vi "DSF.Execution.Runtime.Plugin Manager.Find Plugin Classes.Configuration.vi"(8 "error in (no error)":errorcluster, 10 "Plugin objects":refnum<class>[](array[class]), 11 "Plugin Manager in":refnum<class "DSF.Engine.Runtime.Plugin Manager.lvclass">) -> (0 "error out":errorcluster, 2 "Plugin Configuration Classes":T1, 3 "Plugin Manager out":refnum<class "DSF.Engine.Runtime.Plugin Manager.lvclass">)   [LabVIEW 2016, in "DSF.Engine.lvlib" / "DSF.Engine.Runtime.Plugin Manager.lvclass"]
uses:
  DSF.Engine.Runtime.Plugin Manager.lvclass
  Shared/Typedefs/DSF.Shared.Typedefs.Plugin Classes.Configuration.ctl
  Shared/Classes/Plugin/DSF.Shared.Configuration.Plugin.lvclass
  Shared/Classes/Transfer Group/DSF.Shared.Configuration.Transfer Group.lvclass
  Shared/Classes/Transfer/DSF.Shared.Configuration.Transfer.lvclass
  DSF.Shared.lvlib
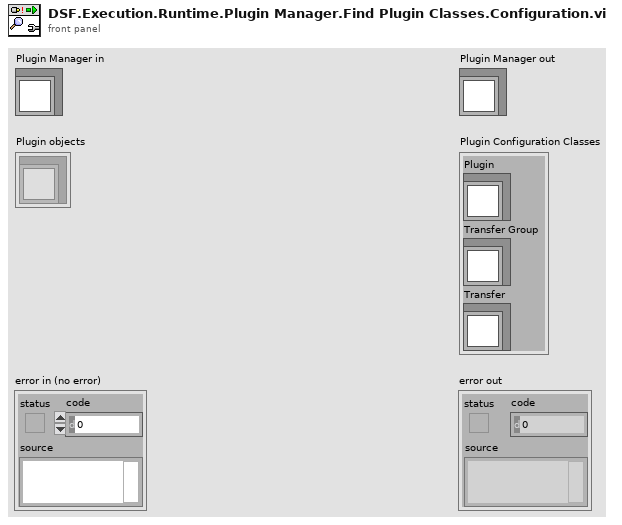
[diagram p1: front panel]
types:
  T1 = typedef "DSF.Shared.lvlib/DSF.Shared.Typedefs.Plugin Classes.Configuration.ctl" = cluster{"Plugin":refnum<class "DSF.Shared.Configuration.Plugin.lvclass">, "Transfer Group":refnum<class "DSF.Shared.Configuration.Transfer Group.lvclass">, "Transfer":refnum<class "DSF.Shared.Configuration.Transfer.lvclass">}
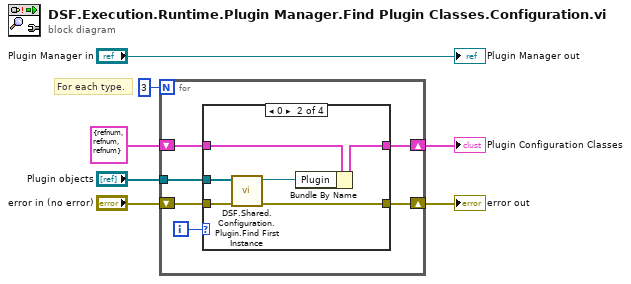
[diagram p0: block diagram]
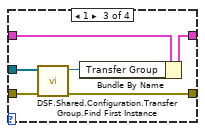
[diagram p3: hidden frame]
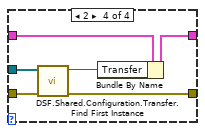
[diagram p4: hidden frame]
diagram:
  # "For each type."
  n1 = for {
    N: 3 -> [_]
    shift-right: [w11] -> w3
    shift-left: T1 {"Plugin"=refnum, "Transfer Group"=refnum, "Transfer"=refnum} ("Configuration") -> [w12]
    shift-right: [w10] -> w2
    shift-left: "error in (no error)" -> [w9]
    tunnel: "Plugin objects" -> [w8]
    i -> [w13]
    n2 = case shown="0" w13 {
      tunnel: w12 -> [w15 w21 w27 w33]
      tunnel: [w15 w20 w26 w32] -> w11
      tunnel: [w14 w18 w23 w29] -> w10
      tunnel: w9 -> [w14 w17 w24 w30]
      tunnel: w8 -> [_ w16 w25 w31]
      frame -1, Default {
      }
      frame 0 {
        n3 = call "DSF.Shared.Configuration.Plugin.Find First Instance.vi"("error in (no error)"=w17, "objects"=w16) -> ("error out"=w18:errorcluster, "Plugin Configuration"=w19:refnum<class "DSF.Shared.Configuration.Plugin.lvclass">)  [unwired: 7 in, 1 out]
        n4 = Bundle By Name(cluster=w21, "Plugin"=w19) -> (w20:T1)
      }
      frame 1 {
        n5 = call "DSF.Shared.Configuration.Transfer Group.Find First Instance.vi"("error in (no error)"=w24, "objects"=w25) -> ("error out"=w23:errorcluster, "Transfer Group Configuration"=w22:refnum<class "DSF.Shared.Configuration.Transfer Group.lvclass">)  [unwired: 7 in, 1 out]
        n6 = Bundle By Name(cluster=w27, "Transfer Group"=w22) -> (w26:T1)
      }
      frame 2 {
        n7 = call "DSF.Shared.Configuration.Transfer.Find First Instance.vi"("error in (no error)"=w30, "objects"=w31) -> ("error out"=w29:errorcluster, "Transfer Configuration"=w28:refnum<class "DSF.Shared.Configuration.Transfer.lvclass">)  [unwired: 7 in, 1 out]
        n8 = Bundle By Name(cluster=w33, "Transfer"=w28) -> (w32:T1)
      }
    }
  }
  "error out" <- w2
  "Plugin Configuration Classes" <- w3
  "Plugin Manager out" <- "Plugin Manager in"
